vi "generate table.vi"(5 "to TEC":refnum<vi>, 6 "Direction":T1(radio), 7 "from TEC":refnum<vi>, 8 "error in":errorcluster, 9 "avail tags":refnum<vi>, 10 "engine configuration in":refnum<class "engine configuration.lvclass">, 11 "TEC in":refnum<class "TEC configuration.lvclass">) -> (0 "error out":errorcluster, 3 "TEC out":refnum<class "TEC configuration.lvclass">)   [LabVIEW 2013, in "TEC editor node.lvclass"]
uses:
  TEC editor node.lvclass
  module/configuration/TEC configuration.lvclass
  <vilib>/NI/Module Execution Interface/Engine Configuration/engine configuration.lvclass
  <vilib>/NI/Tag Bus Module Framework/root configuration/TBM configuration.lvclass/TBM configuration.ctl
  module/configuration/TEC configuration.lvclass/TEC configuration.ctl
  <vilib>/NI/Tag Bus/tag/tag descriptor.lvclass/tag descriptor.ctl
  <vilib>/NI/Tag Bus Module Framework/channel/channel classification.ctl
  <vilib>/NI/Tag Bus Module Framework/channel/TBM channel.lvclass/TBM channel.ctl
  <vilib>/NI/Module Execution Interface/Engine Configuration/engine configuration.lvclass/engine configuration.ctl
  <vilib>/NI/Tag Bus/tag/read tag name.vi
  <vilib>/NI/Tag Bus Module Framework/channel/Read channel classification.vi
  <vilib>/NI/Tag Bus/tag/read data type.vi
  <vilib>/NI/Tag Bus Module Framework/root configuration/Read instance name.vi
  module/configuration/Read channels.vi
  <vilib>/NI/Tag Bus Module Framework/root configuration/create GUID.vi
  <vilib>/NI/Tag Bus Module Framework/channel/TBM channel.lvclass
  <vilib>/NI/Tag Bus/tag/tag descriptor.lvclass
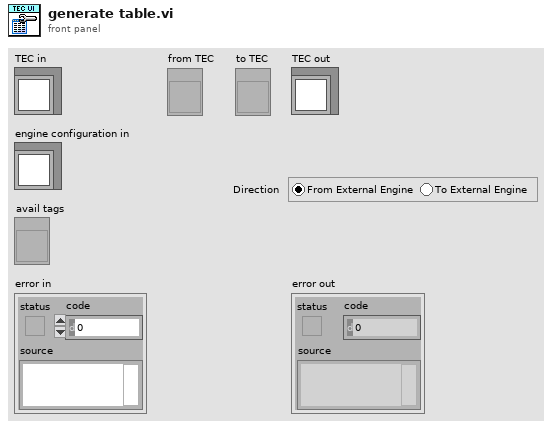
[diagram p1: front panel]
types:
  T1 = enum32{"From External Engine", "To External Engine"}
  T2 = typedef "tag bus.lvlib/tag descriptor.lvclass/Data Type.ctl" = enum16{"Double", "Single", "I64", "I32", "I16", "I8", "U64", "U32", "U16", "U8", "Boolean", "String", "Array of Double", "Array of Single", "Array of I64", "Array of I32", "Array of I16", "Array of I8", "Array of U64", "Array of U32", "Array of U16", "Array of U8", "Array of Boolean", "Array of String"}
  T3 = typedef "TBM channel.lvclass/channel classification.ctl" = enum16{"input data", "output data", "processing parameter", "processing result"}
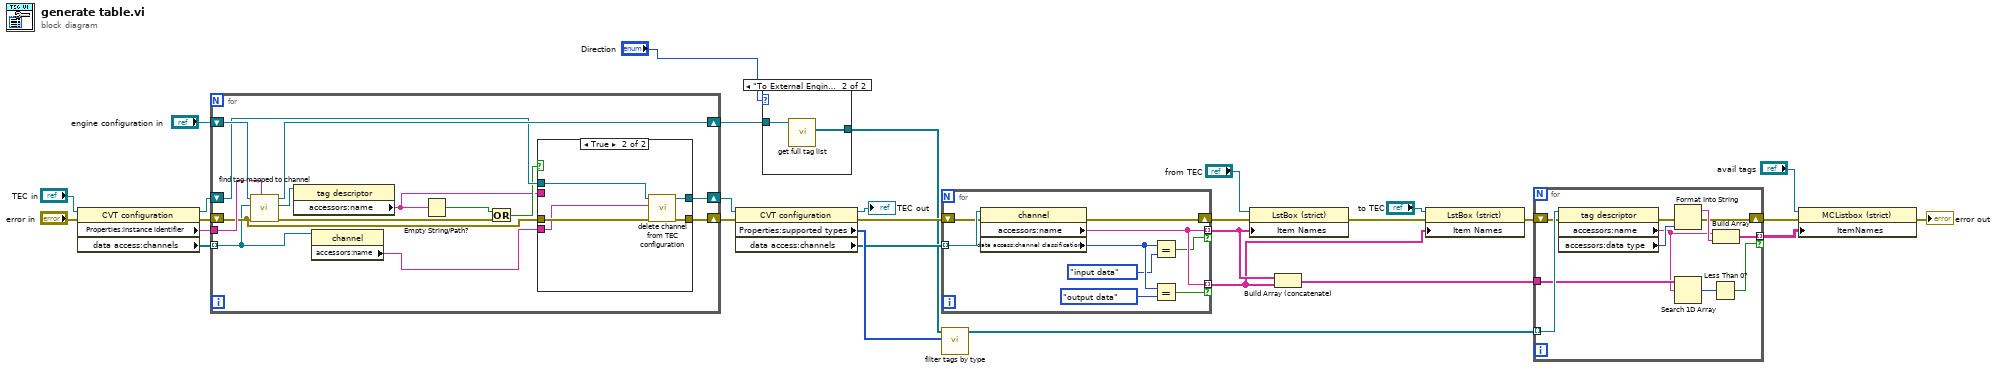
[diagram p0: block diagram]
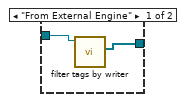
[diagram p2: hidden frame]
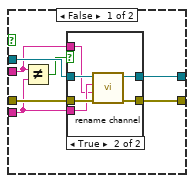
[diagram p3: hidden frame]
diagram:
  n1 = property class="CVT configuration"(reference="TEC in", error in="error in") -> (reference out=w27:refnum<class "TEC configuration.lvclass">, error out=w28:errorcluster, "Properties:instance identifier"=w23:string, "data access:channels"=w29:refnum<class "TBM channel.lvclass">[])
  n2 = for {
    tunnel: w29 -> [w33] mode=indexing
    shift-right: [w41] -> w14
    shift-left: "engine configuration in" -> [w43]
    shift-right: [w38] -> w26
    shift-left: w27 -> [w36]
    tunnel: w23 -> [w42]
    shift-right: [w37] -> w25
    shift-left: w28 -> [w34]
    n3 = call <vilib>:"find tag mapped to channel.vi"("owner"=w42, "error in"=w34, "channel"=w33, "engine configuration in"=w43) -> ("error out"=w32:errorcluster, "tag"=w40:refnum<class "tag descriptor.lvclass">, "engine configuration out"=w41:refnum<class "engine configuration.lvclass">)  [unwired: 5 in]
    n4 = property class="tag descriptor"(reference=w40) -> ("accessors:name"=w30:string)  [unwired: 1 in, 2 out]
    n5 = property class="channel"(reference=w33) -> ("accessors:name"=w31:string)  [unwired: 1 in, 2 out]
    n6 = Empty String/Path?(string/path=w30) -> (empty?=w39:bool)
    n7 = Or(x=w39, y=w32) -> (x .or. y?=w35:bool)
    n8 = case shown="True" w35 {
      tunnel: [w47 w63] -> w38
      tunnel: [w50 w62] -> w37
      tunnel: w34 -> [w49 w61]
      tunnel: w36 -> [w48 w60]
      tunnel: w31 -> [w45 w59]
      tunnel: w30 -> [w44 _]
      frame False {
        n9 = Not Equal?(x=w44, y=w45) -> (x != y?=w46:bool)
        n10 = case shown="True" w46 {
          tunnel: [w52 w57] -> w50
          tunnel: w49 -> [w52 w58]
          tunnel: w48 -> [w51 w56]
          tunnel: [w51 w55] -> w47
          tunnel: w45 -> [_ w54]
          tunnel: w44 -> [_ w53]
          frame False {
          }
          frame True {
            n11 = call "rename channel.vi"("error in"=w58, "new name"=w53, "old name"=w54, "TEC configuration in"=w56) -> ("error out"=w57:errorcluster, "TEC configuration out"=w55:refnum<class "TEC configuration.lvclass">)  [unwired: 6 in]
          }
        }
      }
      frame True {
        n12 = call "delete channel from TEC configuration.vi"("error in"=w61, "channel to delete"=w59, "TEC configuration in"=w60) -> ("error out"=w62:errorcluster, "TEC configuration out"=w63:refnum<class "TEC configuration.lvclass">)  [unwired: 7 in]
      }
    }
  }
  n13 = property class="CVT configuration"(reference=w26, error in=w25) -> (reference out=→"TEC out":refnum<class "TEC configuration.lvclass">, error out=w21:errorcluster, "Properties:supported types"=w24:T2[], "data access:channels"=w22:refnum<class "TBM channel.lvclass">[])
  n14 = case shown="\"To External Engine\"" "Direction" {
    tunnel: w14 -> [w65 w67]
    tunnel: [w64 w66] -> w13
    frame "From External Engine" {
      n15 = call <vilib>:"filter tags by writer.vi"("engine configuration in"=w65) -> ("tag list"=w64:refnum<class "tag descriptor.lvclass">[])  [unwired: 9 in, 1 out]
    }
    frame "To External Engine" {
      n16 = call <vilib>:"get full tag list.vi"("engine configuration in"=w67) -> ("tag list"=w66:refnum<class "tag descriptor.lvclass">[])  [unwired: 9 in, 1 out]
    }
  }
  n17 = for {
    tunnel: w22 -> [w76] mode=indexing
    shift-right: [w75] -> w7
    shift-left: w21 -> [w74]
    tunnel: [w73] -> w3 mode=indexing if=w71
    tunnel: [w73] -> w4 mode=indexing if=w70
    n18 = property class="channel"(reference=w76, error in=w74) -> (error out=w75:errorcluster, "accessors:name"=w73:string, "data access:channel classification"=w72:T3)  [unwired: 1 out]
    n19 = Equal?(x=w72, y=channel_classification."input data") -> (x = y?=w70:bool)
    n20 = Equal?(x=w72, y=channel_classification."output data") -> (x = y?=w71:bool)
  }
  n21 = call <vilib>:"filter tags by type.vi"("allowable types"=w24, "tags in"=w13) -> ("filtered tags"=w20:refnum<class "tag descriptor.lvclass">[])  [unwired: 9 in]
  n22 = property class="LstBox (strict)"(reference="from TEC", error in=w7, "Item Names"=w4) -> (error out=w6:errorcluster)  [unwired: 1 out]
  n23 = Build Array (concatenate)(w4, w3) -> (w2:string[])
  n24 = property class="LstBox (strict)"(reference="to TEC", error in=w6, "Item Names"=w3) -> (error out=w19:errorcluster)  [unwired: 1 out]
  n25 = for {
    tunnel: w20 -> [w85] mode=indexing
    shift-right: [w82] -> w18
    shift-left: w19 -> [w84]
    tunnel: [w81] -> w17 mode=indexing if=w77
    tunnel: w2 -> [w80]
    n26 = property class="tag descriptor"(reference=w85, error in=w84) -> (error out=w83:errorcluster, "accessors:name"=w78:string, "accessors:data type"=w86:T2)  [unwired: 1 out]
    n27 = Format Into String(error in=w83, w86) -> (resulting string=w87:string, error out=w82:errorcluster)  [unwired: 2 in]
    n28 = Search 1D Array(1D array=w80, element=w78) -> (index of element=w79:i32)  [unwired: 1 in]
    n29 = Less Than 0?(x=w79) -> (x < 0?=w77:bool)
    n30 = Build Array(w78, w87) -> (w81:string[])
  }
  n31 = property class="MCListbox (strict)"(reference="avail tags", error in=w18, "ItemNames"=w17) -> (error out=→"error out":errorcluster)  [unwired: 1 out]
